vi "Next State.vi"(8 "error in (no error)":errorcluster, 10 "New_State":u32, 11 "State Machine in":refnum<class "State Machine.lvclass">) -> (0 "error out":errorcluster, 3 "State Machine out":refnum<class "State Machine.lvclass">)   [LabVIEW 2018, in "State Machine.lvclass"]
doc: "Este VI escreve na classe o próximo estado, salvando o estado anterior em \"previous state\"."
uses:
  State Machine.lvclass
  State Machine.lvclass/State Machine.ctl
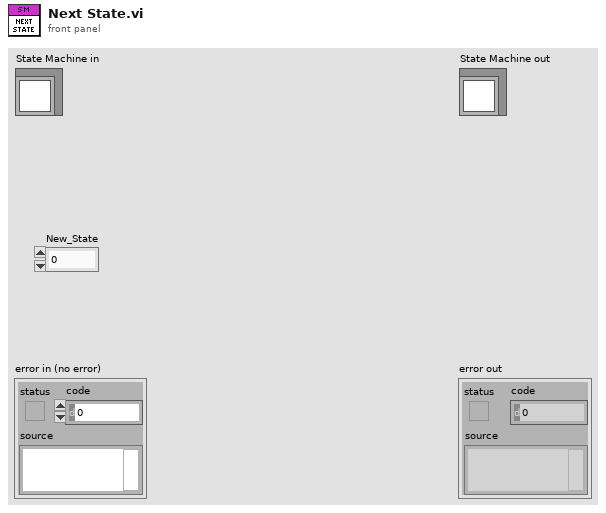
[diagram p1: front panel]
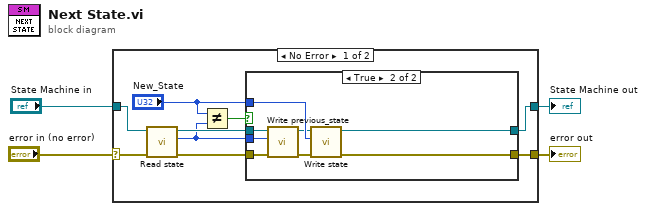
[diagram p0: block diagram]
diagram:
  n1 = case shown="No Error" "error in (no error)" {
    selector: "error in (no error)" -> [w10 w25]
    tunnel: [w11 w25] -> w2
    tunnel: [w13 w24] -> w1
    tunnel: "State Machine in" -> [w8 w24]
    frame No Error {
      n2 = call "Read state.vi"("error in (no error)"=w10, "State Machine in"=w8) -> ("error out"=w9:errorcluster, "state"=w5:u32, "State Machine out"=w7:refnum<class "State Machine.lvclass">)  [unwired: 7 in]
      n3 = Not Equal?(x="New_State", y=w5) -> (x != y?=w12:bool)
      n4 = case shown="True" w12 {
        tunnel: w7 -> [w15 w22]
        tunnel: [w15 w18] -> w13
        tunnel: w5 -> [_ w23]
        tunnel: "New_State" -> [_ w20]
        tunnel: [w14 w19] -> w11
        tunnel: w9 -> [w14 w17]
        frame False {
          # "ESTADO DESEJADO JÁ É O ESTADO ATUAL"
        }
        frame True {
          n5 = call "Write previous_state.vi"("error in (no error)"=w17, "previous_state"=w23, "State Machine in"=w22) -> ("error out"=w21:errorcluster, "State Machine out"=w16:refnum<class "State Machine.lvclass">)  [unwired: 7 in]
          n6 = call "Write state.vi"("error in (no error)"=w21, "state"=w20, "State Machine in"=w16) -> ("error out"=w19:errorcluster, "State Machine out"=w18:refnum<class "State Machine.lvclass">)  [unwired: 7 in]
        }
      }
    }
    frame Error {
    }
  }
  "error out" <- w2
  "State Machine out" <- w1
